vi "Offset.vi"(7 "Raw Data Waveform":T1, 10 "Offset":i32, 11 "(Index_Pointer)":refnum<class "Absolute_Pointer.lvclass">) -> (3 "(Index_Pointer) Out":refnum<class "Absolute_Pointer.lvclass">)   [LabVIEW 2020, in "Absolute_Pointer.lvclass"]
uses:
  Absolute_Pointer.lvclass
  Universal Controls/Waveform_Data.ctl
  Absolute_Pointer.lvclass/Absolute_Pointer.ctl
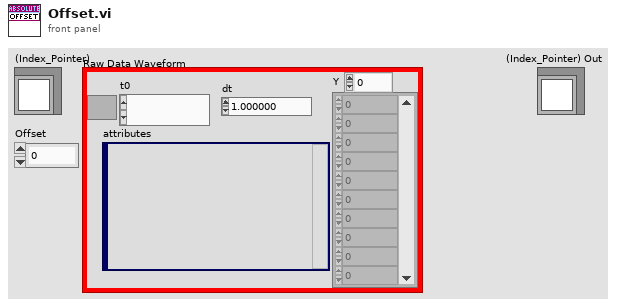
[diagram p1: front panel]
types:
  T1 = typedef "Waveform_Data.ctl" = waveform(dbl)
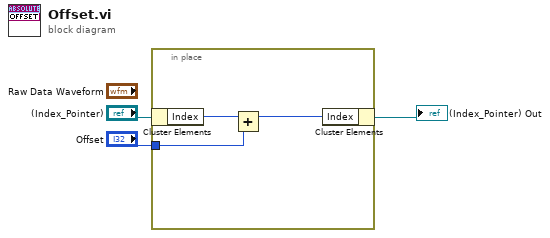
[diagram p0: block diagram]
diagram:
  n1 = in-place {
    in-place-border: "Offset" -> [w4]
    n2 = in-place-cluster #1("(Index_Pointer)") -> ("Index"=w6:i32)
    n3 = Add(x=w6, y=w4) -> (x+y=w5:i32)
    n4 = in-place-cluster #1("Index"=w5) -> (→"(Index_Pointer) Out":refnum<class "Absolute_Pointer.lvclass">)
  }
